vi "Run.vi"(7 "Type y_true":T1(ring), 8 "error in (no error)":errorcluster caption="entrée d'erreur (pas d'erreur)", 9 "y_score":string[][](array[string]), 10 "y_true":string[][](array[string]), 11 "Label_Ranking_Average_PS en entrée":refnum<class "Label_Ranking_Average_PS.lvclass">) -> (0 "error out":errorcluster caption="sortie d'erreur", 2 "String Data":string, 3 "Label_Ranking_Average_PS en entrée":refnum<class "Label_Ranking_Average_PS.lvclass">)   [LabVIEW 2020, in "Label_Ranking_Average_PS.lvclass"]
doc: "Returns : \n\n- score : float"
uses:
  Label_Ranking_Average_PS.lvclass
  Label_Ranking_Average_PS.lvclass/Label_Ranking_Average_PS.ctl
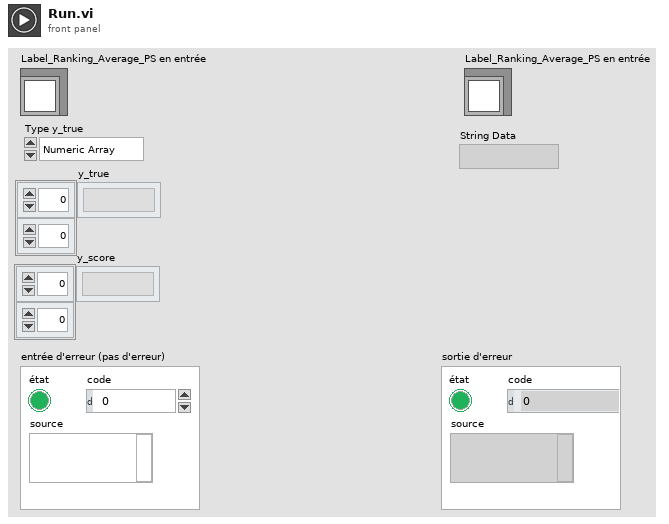
[diagram p1: front panel]
types:
  T1 = enum16{"Numeric Array", "String Array", "Sparse"}
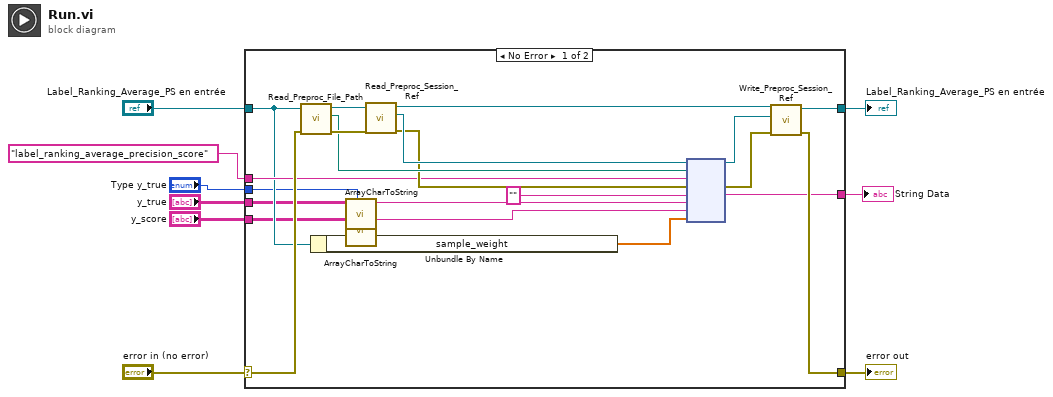
[diagram p0: block diagram]
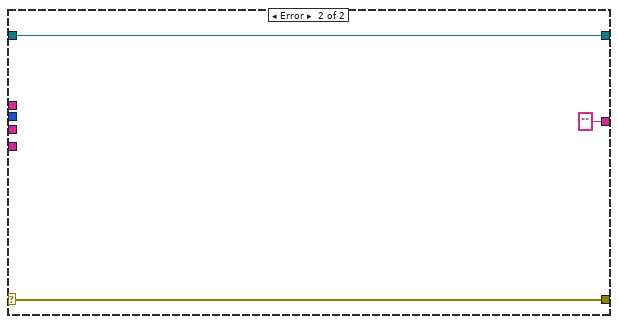
[diagram p2: hidden frame]
diagram:
  n1 = case shown="No Error" "error in (no error)" {
    selector: "error in (no error)" -> [w19 w33]
    tunnel: [w20 w33] -> w8
    tunnel: [w21 w32] -> w6
    tunnel: "Label_Ranking_Average_PS en entrée" -> [w16 w32]
    tunnel: "label_ranking_average_precision_score" -> [w18 _]
    tunnel: [w17 ""] -> w5
    tunnel: "y_true" -> [w14 _]
    tunnel: "y_score" -> [w11 _]
    tunnel: "Type y_true" -> [w10 _]
    frame No Error {
      n2 = call-dynamic "Read_Preproc_File_Path.vi"("error in (no error)"=w19, "Python in"=w16) -> ("error out"=w29:errorcluster, "File_Path"=w28:path, "Python out"=w30:refnum<class "Label_Ranking_Average_PS.lvclass">)  [unwired: 7 in]
      n3 = Unbundle By Name(w16) -> ("sample_weight"=w15:dbl[])
      n4 = call "ArrayCharToString.vi"("Type"=w10, "TAB"=w14) -> ("Instruction"=w13:string)  [unwired: 9 in]
      n5 = call "ArrayCharToString.vi"("TAB"=w11) -> ("Instruction"=w12:string)  [unwired: 10 in]
      n6 = call-dynamic "Read_Preproc_Session_Ref.vi"("error in (no error)"=w29, "Python in"=w30) -> ("error out"=w26:errorcluster, "Session_ref"=w27:refnum<k35>, "Python out"=w25:refnum<class "Label_Ranking_Average_PS.lvclass">)  [unwired: 7 in]
      n7 = node(w27, w28, w18, w26, "", w13, w12, w15) -> (w23:refnum<k35>, w24:errorcluster, w17:string)  [unwired: 3 in, 2 out]
      n8 = call-dynamic "Write_Preproc_Session_Ref.vi"("error in (no error)"=w24, "Session_ref"=w23, "Python in"=w25) -> ("error out"=w20:errorcluster, "Python out"=w21:refnum<class "Label_Ranking_Average_PS.lvclass">)  [unwired: 7 in]
    }
    frame Error {
    }
  }
  "error out" <- w8
  "Label_Ranking_Average_PS en entrée" <- w6
  "String Data" <- w5
